vi "GetCurrent.vi"(8 "Error In":errorcluster, 11 "object in":refnum<class "IEnumerator.lvclass">) -> (0 "Error Out":errorcluster, 2 "property":bool, 3 "object out":refnum<class "IEnumerator.lvclass">)   [LabVIEW 2020, in "IEnumerator.lvclass"]
uses:
  IEnumerator.lvclass
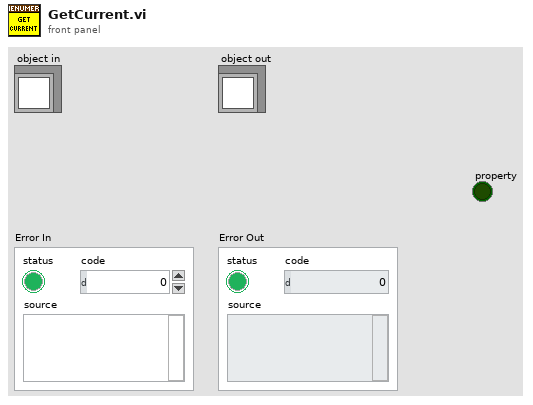
[diagram p1: front panel]
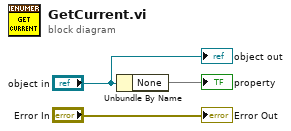
[diagram p0: block diagram]
diagram:
  n1 = Unbundle By Name("object in") -> ("None"=→"property")
  "Error Out" <- "Error In"
  "object out" <- "object in"
